vi "Hauptprogramm.vi"() -> ()   [LabVIEW 2021]
uses:
  Agilent E364X Series/Agilent E364X Series.lvlib
panel:
  out "Spannung (V)":dbl
  in  "Ausgang auswählen":string(combo)="OUT1"
  in  "Ausgang am Ende ausschalten":bool
  in  "Ausgang anschalten":bool
  in  "Agilent E3646A Name":refnum<visa-resource-name>="GPIB0::5::INSTR"
  in  "Maximale Spannung (20 V)":dbl=22.0 format="%.2p"
  in  "Maximale Stromstärke (1.5 A)":dbl format="%.2p"
  out "Schleifendurchlauf":i32
  out "Zwischenspeicher des Arduino":string
  in  "Programm stopen":bool
  out "Abstand (mm)":dbl
  in  "Byte-Anzahl":u32=11
  in  "Arduino Name":refnum<visa-resource-name>="COM3"
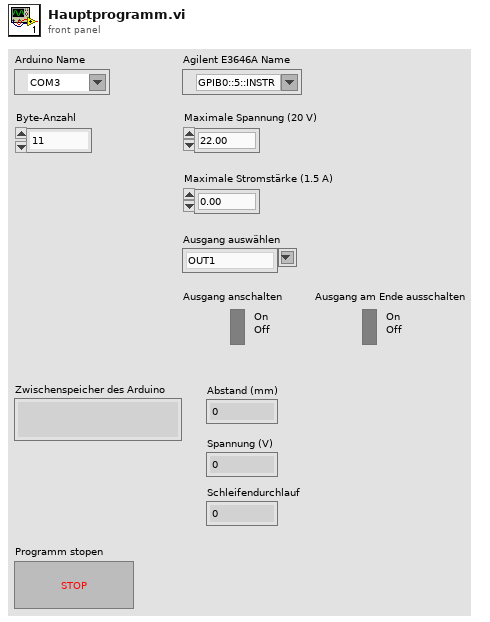
[diagram p1: front panel]
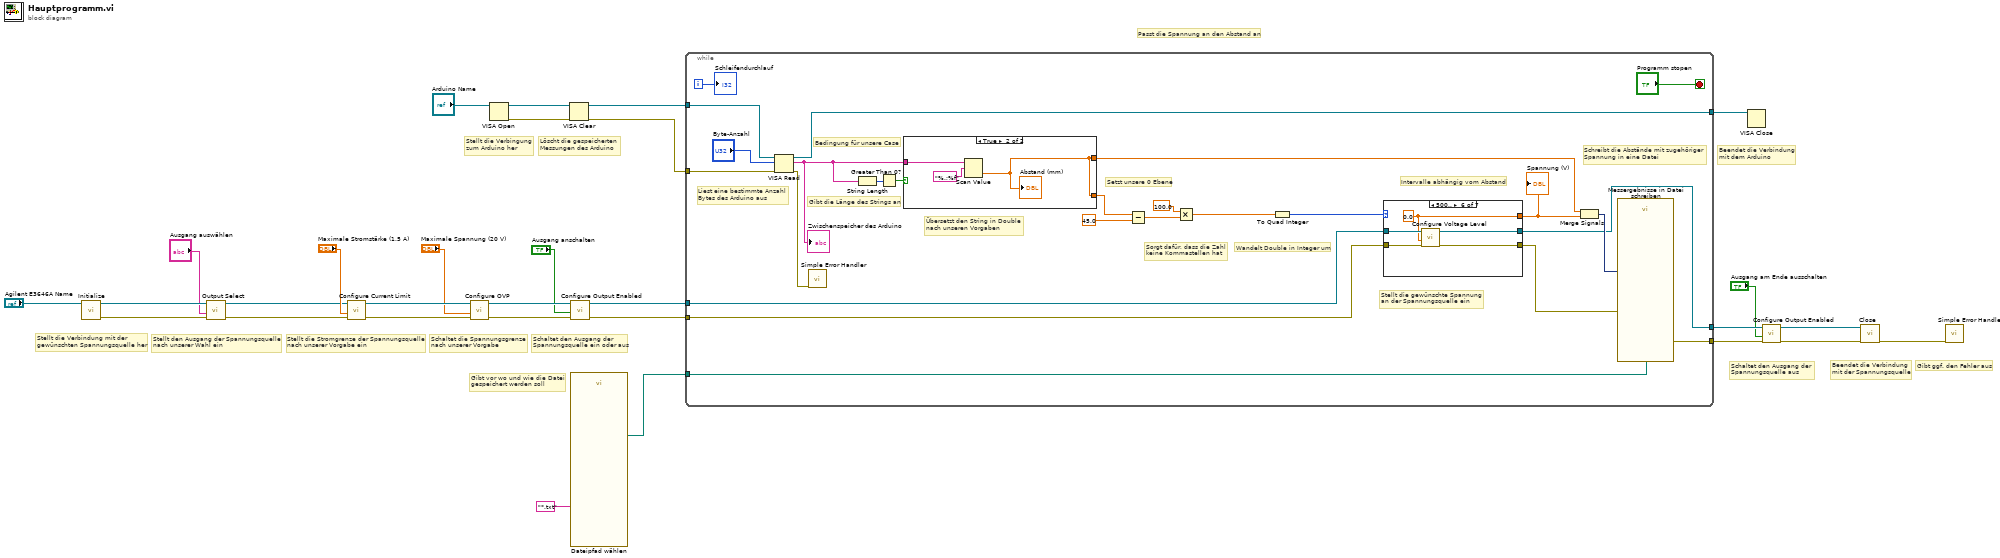
[diagram p0: block diagram]
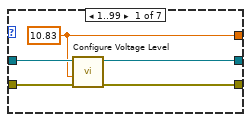
[diagram p2: hidden frame]
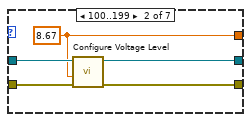
[diagram p3: hidden frame]
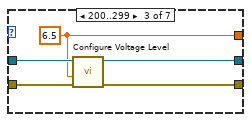
[diagram p4: hidden frame]
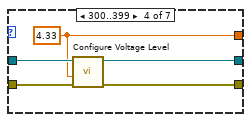
[diagram p5: hidden frame]
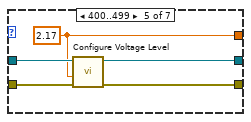
[diagram p6: hidden frame]
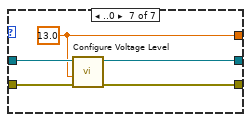
[diagram p7: hidden frame]
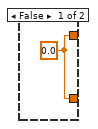
[diagram p8: hidden frame]
diagram:
  # "Passt die Spannung an den Abstand an"
  # "Gibt ggf. den Fehler aus"
  # "Beendet die Verbindung \nmit der Spannungsquelle"
  # "Schaltet den Ausgang der \nSpannungsquelle aus"
  # "Beendet die Verbindung\nmit dem Arduino"
  # "Löscht die gespeicherten \nMessungen des Arduino"
  # "Stellt die Verbingung \nzum Arduino her"
  # "Gibt vor wo und wie die Datei \ngespeichert werden soll"
  # "Stellt die Verbindung mit der \ngewünschten Spannungsquelle her"
  # "Schaltet den Ausgang der \nSpannungsquelle ein oder aus"
  # "Schaltet die Spannungsgrenze \nnach unserer Vorgabe"
  # "Stellt die Stromgrenze der Spannungsquelle \nnach unserer Vorgabe ein"
  # "Stellt den Ausgang der Spannungsquelle \nnach unserer Wahl ein"
  n1 = call "Initialize.vi"("VISA resource name"="Agilent E3646A Name") -> ("error out"=w19:errorcluster, "VISA resource name out"=w20:refnum<visa-resource-name>)  [unwired: 9 in]
  n2 = call "Output Select.vi"("error in (no error)"=w19, "Instrument Select (Output 1)"="Ausgang auswählen", "VISA resource name"=w20) -> ("error out"=w22:errorcluster, "VISA resource name out"=w23:refnum<visa-resource-name>)  [unwired: 7 in]
  n3 = call "Configure Current Limit.vi"("error in (no error)"=w22, "Current Limit (0.0 Amps)"="Maximale Stromstärke (1.5 A)", "VISA resource name"=w23) -> ("error out"=w25:errorcluster, "VISA resource name out"=w8:refnum<visa-resource-name>)  [unwired: 7 in]
  n4 = call "Configure OVP.vi"("error in (no error)"=w25, "Limit (22.0 Volts)"="Maximale Spannung (20 V)", "VISA resource name"=w8) -> ("error out"=w17:errorcluster, "VISA resource name out"=w16:refnum<visa-resource-name>)  [unwired: 7 in]
  n5 = VISA Open(VISA resource name="Arduino Name") -> (VISA resource name=w28:refnum<visa-resource-name>, error out=w26:errorcluster)  [unwired: 4 in]
  n6 = VISA Clear(VISA resource name=w28, error in (no error)=w26) -> (VISA resource name out=w27:refnum<visa-resource-name>, error out=w5:errorcluster)
  n7 = call "Configure Output Enabled.vi"("error in (no error)"=w17, "Output Enabled (F: Off)"="Ausgang anschalten", "VISA resource name"=w16) -> ("error out"=w10:errorcluster, "VISA resource name out"=w11:refnum<visa-resource-name>)  [unwired: 7 in]
  n8 = call "Dateipfad wählen"("pattern (all files)"="*.txt") -> ("selected path"=w15:path)  [unwired: 11 in, 3 out]
  n9 = while {
    tunnel: w27 -> [w50]
    tunnel: w5 -> [w54]
    tunnel: w11 -> [w47]
    tunnel: [w31] -> w14
    tunnel: w10 -> [w32]
    tunnel: w15 -> [w42]
    tunnel: [w38] -> w12
    tunnel: [w34] -> w9
    i -> [w36]
    stop <- "Programm stopen" stop-if-true
    # "Bedingung für unsere Case"
    # "Gibt die Länge des Strings an"
    # "Schreibt die Abstände mit zugehöriger \nSpannung in eine Datei"
    # "Intervalle abhängig vom Abstand"
    # "Stellt die gewünschte Spannung \nan der Spannungsquelle ein"
    # "Wandelt Double in Integer um"
    # "Setzt unsere 0 Ebene"
    # "Sorgt dafür, dass die Zahl \nkeine Kommastellen hat"
    # "Übersetzt den String in Double \nnach unseren Vorgaben"
    # "Liest eine bestimmte Anzahl \nBytes des Arduino aus"
    n10 = VISA Read(VISA resource name=w50, byte count="Byte-Anzahl", error in (no error)=w54) -> (VISA resource name out=w34:refnum<visa-resource-name>, read buffer=w35:string, error out=w30:errorcluster)  [unwired: 1 out]
    "Zwischenspeicher des Arduino" <- w35
    n11 = call <vilib>:"Simple Error Handler.vi"("error in (no error)"=w30) -> ()  [unwired: 4 in, 5 out]
    n12 = String Length(string=w35) -> (length=w52:i32)
    n13 = Greater Than 0?(x=w52) -> (x > 0?=w51:bool)
    n14 = case shown="True" w51 {
      tunnel: w35 -> [_ w92]
      tunnel: [w90 w91] -> w48
      tunnel: [w90 w91] -> w41
      frame False {
        w90 = 0.0
      }
      frame True {
        n15 = Scan Value(string=w92, format string="%.;%f") -> (value=w91:dbl)  [unwired: 1 in, 1 out]
        "Abstand (mm)" <- w91
      }
    }
    n16 = Subtract(x=w48, y=45.0) -> (x-y=w46:dbl)
    n17 = Multiply(x=100.0, y=w46) -> (x*y=w44:dbl)
    n18 = To Quad Integer(1:w44) -> (0:w43:i64)
    n19 = case shown="500.." w43 {
      tunnel: w32 -> [w59 w64 w69 w74 w79 w84 w89]
      tunnel: w47 -> [w57 w62 w67 w72 w77 w82 w87]
      tunnel: [w58 w63 w68 w73 w78 w83 w88] -> w39
      tunnel: [w56 w61 w66 w71 w76 w81 w86] -> w31
      tunnel: [w55 w60 w65 w70 w75 w80 w85] -> w40
      frame 1..99 {
        w55 = 10.83
        n20 = call "Configure Voltage Level.vi"("error in (no error)"=w59, "Level (0.0 Volts)"=w55, "VISA resource name"=w57) -> ("error out"=w58:errorcluster, "VISA resource name out"=w56:refnum<visa-resource-name>)  [unwired: 7 in]
      }
      frame 100..199 {
        w60 = 8.67
        n21 = call "Configure Voltage Level.vi"("error in (no error)"=w64, "Level (0.0 Volts)"=w60, "VISA resource name"=w62) -> ("error out"=w63:errorcluster, "VISA resource name out"=w61:refnum<visa-resource-name>)  [unwired: 7 in]
      }
      frame 200..299 {
        w65 = 6.5
        n22 = call "Configure Voltage Level.vi"("error in (no error)"=w69, "Level (0.0 Volts)"=w65, "VISA resource name"=w67) -> ("error out"=w68:errorcluster, "VISA resource name out"=w66:refnum<visa-resource-name>)  [unwired: 7 in]
      }
      frame 300..399 {
        w70 = 4.33
        n23 = call "Configure Voltage Level.vi"("error in (no error)"=w74, "Level (0.0 Volts)"=w70, "VISA resource name"=w72) -> ("error out"=w73:errorcluster, "VISA resource name out"=w71:refnum<visa-resource-name>)  [unwired: 7 in]
      }
      frame 400..499 {
        w75 = 2.17
        n24 = call "Configure Voltage Level.vi"("error in (no error)"=w79, "Level (0.0 Volts)"=w75, "VISA resource name"=w77) -> ("error out"=w78:errorcluster, "VISA resource name out"=w76:refnum<visa-resource-name>)  [unwired: 7 in]
      }
      frame 500.. {
        w80 = 0.0
        n25 = call "Configure Voltage Level.vi"("error in (no error)"=w84, "Level (0.0 Volts)"=w80, "VISA resource name"=w82) -> ("error out"=w83:errorcluster, "VISA resource name out"=w81:refnum<visa-resource-name>)  [unwired: 7 in]
      }
      frame ..0 {
        w85 = 13.0
        n26 = call "Configure Voltage Level.vi"("error in (no error)"=w89, "Level (0.0 Volts)"=w85, "VISA resource name"=w87) -> ("error out"=w88:errorcluster, "VISA resource name out"=w86:refnum<visa-resource-name>)  [unwired: 7 in]
      }
    }
    "Spannung (V)" <- w40
    n27 = Merge Signals(w41, w40) -> (w37:dynamicdata)
    n28 = call "Messergebnisse in Datei schreiben"("Signals"=w37, "error in (no error)"=w39, "Filename"=w42) -> ("error out"=w38:errorcluster)  [unwired: 14 in, 2 out]
    "Schleifendurchlauf" <- w36
  }
  n29 = VISA Close(VISA resource name=w9) -> ()  [unwired: 1 in, 1 out]
  n30 = call "Configure Output Enabled.vi"("error in (no error)"=w12, "Output Enabled (F: Off)"="Ausgang am Ende ausschalten", "VISA resource name"=w14) -> ("error out"=w1:errorcluster, "VISA resource name out"=w2:refnum<visa-resource-name>)  [unwired: 7 in]
  n31 = call "Close.vi"("error in (no error)"=w1, "VISA resource name"=w2) -> ("error out"=w18:errorcluster)  [unwired: 9 in]
  n32 = call <vilib>:"Simple Error Handler.vi"("error in (no error)"=w18) -> ()  [unwired: 4 in, 5 out]
